vi "Build Message Configuration.vi"(7 "Virtual Memory Unit in":refnum<class "Virtual Memory Unit.lvclass">, 8 "error in (no error)":errorcluster, 10 "Starting Address":u16 format="%04x", 11 "RT-RT Message in":refnum<class "RT-RT Message.lvclass">) -> (0 "error out":errorcluster, 2 "Next Available Address":u16 format="%04x", 3 "RT-RT Message out":refnum<class "RT-RT Message.lvclass">, 5 "Virtual Memory Unit out":refnum<class "Virtual Memory Unit.lvclass">)   [LabVIEW 2020, in "BCI-1553 API.lvlib" / "RT-RT Message.lvclass"]
doc: "Builds the message control and status blocks. Regardless of message type, this block should always be 16 registers long."
uses:
  RT-RT Message.lvclass
  Dependencies/Virtual Memory Unit/Virtual Memory Unit.lvclass
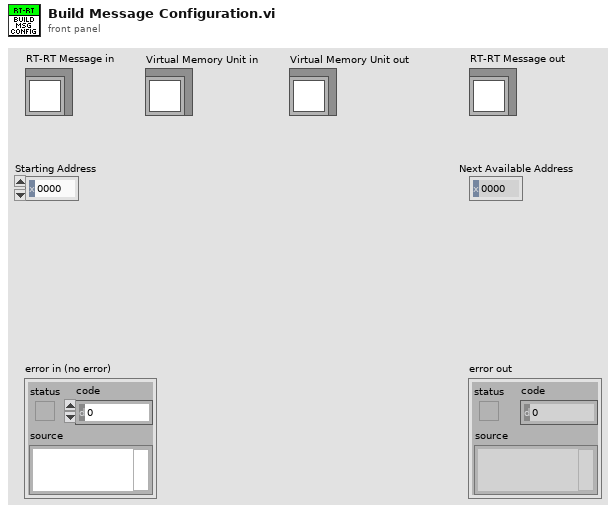
[diagram p1: front panel]
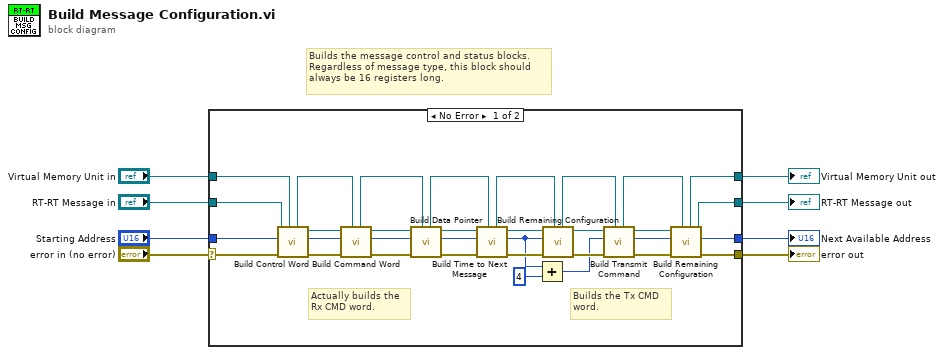
[diagram p0: block diagram]
diagram:
  # "Builds the message control and status blocks.\nRegardless of message type, this block should\nalways be 16 registers long."
  n1 = case shown="No Error" "error in (no error)" {
    selector: "error in (no error)" -> [w41 w45]
    tunnel: [w10 w45] -> w3
    tunnel: [w15 w44] -> w6
    tunnel: "RT-RT Message in" -> [w40 w44]
    tunnel: "Starting Address" -> [w38 w43]
    tunnel: "Virtual Memory Unit in" -> [w39 w42]
    tunnel: [w9 w43] -> w4
    tunnel: [w12 w42] -> w7
    frame No Error {
      # "Builds the Tx CMD\nword."
      # "Actually builds the\nRx CMD word."
      n2 = call-dynamic "Build Control Word.vi"("Virtual Memory Unit in"=w39, "error in (no error)"=w41, "Starting Address"=w38, "Message in"=w40) -> ("error out"=w35:errorcluster, "Next Available Address"=w34:u16, "Message out"=w36:refnum<class "RT-RT Message.lvclass">, "Virtual Memory Unit out"=w37:refnum<class "Virtual Memory Unit.lvclass">)  [unwired: 4 in]
      n3 = call-dynamic "Build Command Word.vi"("Virtual Memory Unit in"=w37, "error in (no error)"=w35, "Starting Address"=w34, "Message in"=w36) -> ("error out"=w23:errorcluster, "Next Available Address"=w25:u16, "Message out"=w26:refnum<class "RT-RT Message.lvclass">, "Virtual Memory Unit out"=w33:refnum<class "Virtual Memory Unit.lvclass">)  [unwired: 4 in]
      n4 = call-dynamic "Build Data Pointer.vi"("Virtual Memory Unit in"=w33, "error in (no error)"=w23, "Starting Address"=w25, "Message in"=w26) -> ("error out"=w30:errorcluster, "Next Available Address"=w31:u16, "Message out"=w32:refnum<class "RT-RT Message.lvclass">, "Virtual Memory Unit out"=w29:refnum<class "Virtual Memory Unit.lvclass">)  [unwired: 4 in]
      n5 = call-dynamic "Build Time to Next Message.vi"("Virtual Memory Unit in"=w29, "error in (no error)"=w30, "Starting Address"=w31, "Message in"=w32) -> ("error out"=w24:errorcluster, "Next Available Address"=w19:u16, "Message out"=w28:refnum<class "RT-RT Message.lvclass">, "Virtual Memory Unit out"=w27:refnum<class "Virtual Memory Unit.lvclass">)  [unwired: 4 in]
      n6 = Add(x=w19, y=u16 4) -> (x+y=w17:u16)
      n7 = call-dynamic "Build Remaining Configuration.vi"("Virtual Memory Unit in"=w27, "error in (no error)"=w24, "Starting Address"=w19, "Message in"=w28) -> ("error out"=w20:errorcluster, "Message out"=w21:refnum<class "RT-RT Message.lvclass">, "Virtual Memory Unit out"=w22:refnum<class "Virtual Memory Unit.lvclass">)  [unwired: 4 in, 1 out]
      n8 = call-dynamic "Build Transmit Command.vi"("Virtual Memory Unit in"=w22, "error in (no error)"=w20, "Starting Address"=w17, "RT-RT Message in"=w21) -> ("error out"=w11:errorcluster, "Next Available Address"=w14:u16, "RT-RT Message out"=w16:refnum<class "RT-RT Message.lvclass">, "Virtual Memory Unit out"=w13:refnum<class "Virtual Memory Unit.lvclass">)  [unwired: 4 in]
      n9 = call-dynamic "Build Remaining Configuration.vi"("Virtual Memory Unit in"=w13, "error in (no error)"=w11, "Starting Address"=w14, "Message in"=w16) -> ("error out"=w10:errorcluster, "Next Available Address"=w9:u16, "Message out"=w15:refnum<class "RT-RT Message.lvclass">, "Virtual Memory Unit out"=w12:refnum<class "Virtual Memory Unit.lvclass">)  [unwired: 4 in]
    }
    frame Error {
    }
  }
  "error out" <- w3
  "RT-RT Message out" <- w6
  "Virtual Memory Unit out" <- w7
  "Next Available Address" <- w4
